vi "Delete Profile.vi"(6 "wait for reply (T)":bool=TRUE, 8 "error in":errorcluster, 10 "Name":string) -> (0 "error out":errorcluster, 1 "timed out?":bool)   [LabVIEW 2025, in "TS Environment Manager.lvlib"]
doc: "Deletes the specified profile from the current file.\n\n_____\nCreated using DQMH Framework: Event Scripter 7.1.1.1528."
uses:
  TS Environment Manager.lvlib
  Delete Profile Argument--cluster.ctl
  Delete Profile (Reply Payload)--cluster.ctl
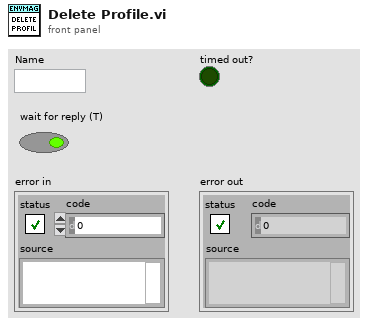
[diagram p1: front panel]
types:
  T1 = typedef "TS Environment Manager.lvlib/Delete Profile Argument--cluster.ctl" = cluster{"Name":string, "Wait Notifier":refnum<notifier>, "wait for reply":bool}
  T2 = typedef "TS Environment Manager.lvlib/Request Events--cluster.ctl" = cluster{"Stop Module":refnum<user-event>, "Show Panel":refnum<user-event>, "Hide Panel":refnum<user-event>, "Get Module Execution Status":refnum<user-event>, "Show Diagram":refnum<user-event>, "Get Installations":refnum<user-event>, "Private.Get Profiles File":refnum<user-event>, "Launch Sequence Editor":refnum<user-event>, "Activate Version":refnum<user-event>, "Add Profile":refnum<user-event>, "Get Profile(s)":refnum<user-event>, "Delete Profile":refnum<user-event>, "Set Profiles File":refnum<user-event>}
  T3 = typedef "TS Environment Manager.lvlib/Delete Profile (Reply Payload)--cluster.ctl" = cluster{"error":errorcluster}
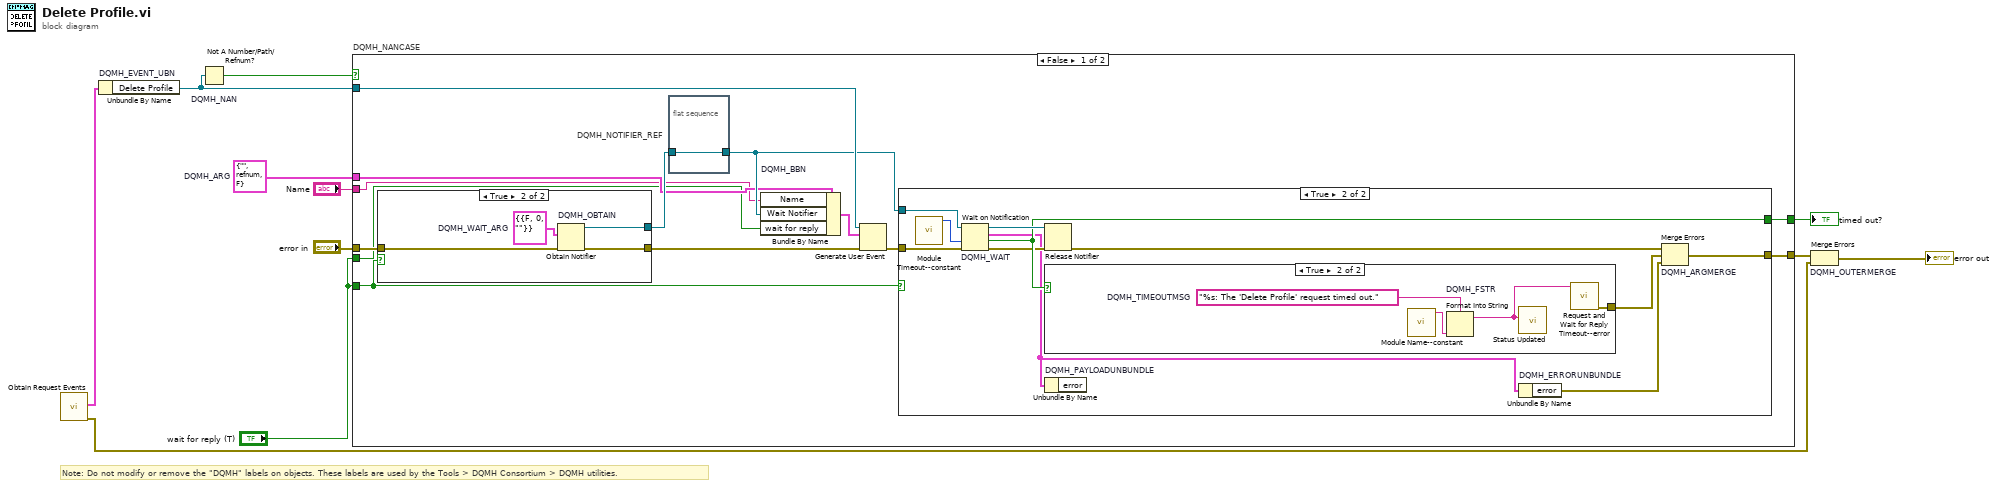
[diagram p0: block diagram]
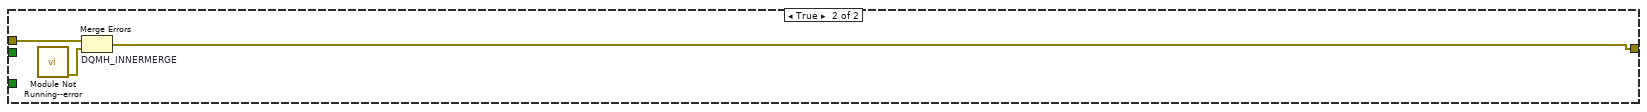
[diagram p5: hidden frame]
diagram:
  w5 = T1 {"Name"="", "Wait Notifier"=refnum, "wait for reply"=FALSE}  # DQMH_ARG
  # "Note: Do not modify or remove the \"DQMH\" labels on objects. These labels are used by the Tools > DQMH Consortium > DQMH utilities."
  n1 = call "Obtain Request Events.vi"() -> ("error out"=w2:errorcluster, "TS Environment Manager Request Events"=w1:T2)  [unwired: 10 in]
  n2 = Unbundle By Name "DQMH_EVENT_UBN"(w1) -> ("Delete Profile"=w6:refnum<user-event>)
  n3 = Not A Number/Path/Refnum? "DQMH_NAN"(number/path/refnum=w6) -> (NaN/Path/Refnum?=w7:bool)
  n4 = case "DQMH_NANCASE" shown="False" w7 {
    tunnel: "error in" -> [w24 w49]
    tunnel: w6 -> [w22 _]
    tunnel: [w19 w48] -> w8
    tunnel: [w20 _] -> w10
    tunnel: "wait for reply (T)" -> [w17 _]
    tunnel: w5 -> [w14 _]
    tunnel: "Name" -> [w13 _]
    tunnel: "wait for reply (T)" -> [w12 _]
    frame False {
      n5 = case shown="True" w17 {
        tunnel: w24 -> [w42 w46]
        tunnel: [w42 w45] -> w21
        tunnel: [_ w43] -> w16
        frame False {
        }
        frame True {
          w44 = T3 {"error"={"status"=FALSE, "code"=0, "source"=""}}  # DQMH_WAIT_ARG
          n6 = Obtain Notifier "DQMH_OBTAIN"(notification data type=w44, error in (no error)=w46) -> (notifier out=w43:refnum<notifier>, error out=w45:errorcluster)  [unwired: 2 in, 1 out]
        }
      }
      n7 = flat-sequence "DQMH_NOTIFIER_REF" {
        tunnel: w16 -> [w25]
        tunnel: [w25] -> w15
        frame #0 {
        }
      }
      n8 = Bundle By Name "DQMH_BBN"(cluster=w14, "Name"=w13, "Wait Notifier"=w15, "wait for reply"=w12) -> (w18:T1)
      n9 = Generate User Event(user event=w22, event data cluster=w18, error in=w21) -> (error out=w23:errorcluster)  [unwired: 1 in, 1 out]
      n10 = case shown="True" w17 {
        tunnel: w23 -> [w26 w37]
        tunnel: w15 -> [_ w36]
        tunnel: [_ w34] -> w20
        tunnel: [w26 w33] -> w19
        frame False {
        }
        frame True {
          n11 = call "Module Timeout--constant.vi"() -> ("Module Timeout"=w27:i32)  [unwired: 11 in]
          n12 = Wait on Notification "DQMH_WAIT"(notifier=w36, timeout in ms (-1)=w27, error in (no error)=w37) -> (notifier out=w35:refnum<notifier>, notification=w28:T3, timed out?=w34:bool, error out=w32:errorcluster)  [unwired: 1 in]
          n13 = Release Notifier(notifier=w35, error in (no error)=w32) -> (error out=w31:errorcluster)  [unwired: 1 in, 2 out]
          n14 = case shown="True" w34 {
            tunnel: [_ w39] -> w29
            frame False {
            }
            frame True {
              w41 = "%s: The 'Delete Profile' request timed out."  # DQMH_TIMEOUTMSG
              n15 = call "Module Name--constant.vi"() -> ("Module Name"=w38:string)  [unwired: 11 in]
              n16 = Format Into String "DQMH_FSTR"(format string=w41, w38) -> (resulting string=w40:string)  [unwired: 2 in, 1 out]
              n17 = call "Status Updated.vi"("Status"=w40) -> ()  [unwired: 10 in, 1 out]
              n18 = call "Request and Wait for Reply Timeout--error.vi"("Error Message"=w40) -> ("error out"=w39:errorcluster)  [unwired: 10 in]
            }
          }
          n19 = Unbundle By Name "DQMH_PAYLOADUNBUNDLE"(w28) -> ()  [unwired: 1 out]
          n20 = Unbundle By Name "DQMH_ERRORUNBUNDLE"(w28) -> ("error"=w30:errorcluster)
          n21 = Merge Errors "DQMH_ARGMERGE"(w31, w29, w30) -> (w33:errorcluster)
        }
      }
    }
    frame True {
      n22 = call "Module Not Running--error.vi"() -> ("error out"=w47:errorcluster)  [unwired: 11 in]
      n23 = Merge Errors "DQMH_INNERMERGE"(w49, w47) -> (w48:errorcluster)
    }
  }
  "timed out?" <- w10
  n24 = Merge Errors "DQMH_OUTERMERGE"(w8, w2) -> (→"error out":errorcluster)
